vi "CityPinYin.vi"() -> ()   [LabVIEW 2017]
panel:
  out "字符串":string
  out "元素":i32
  out "数组":string[][](array[string])
  out "数据":string
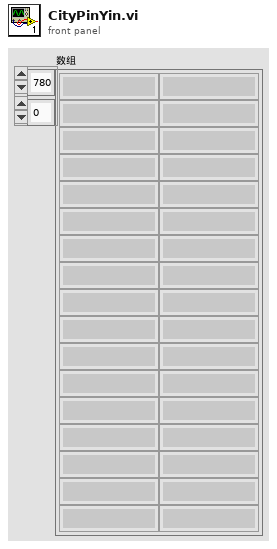
[diagram p1: front panel]
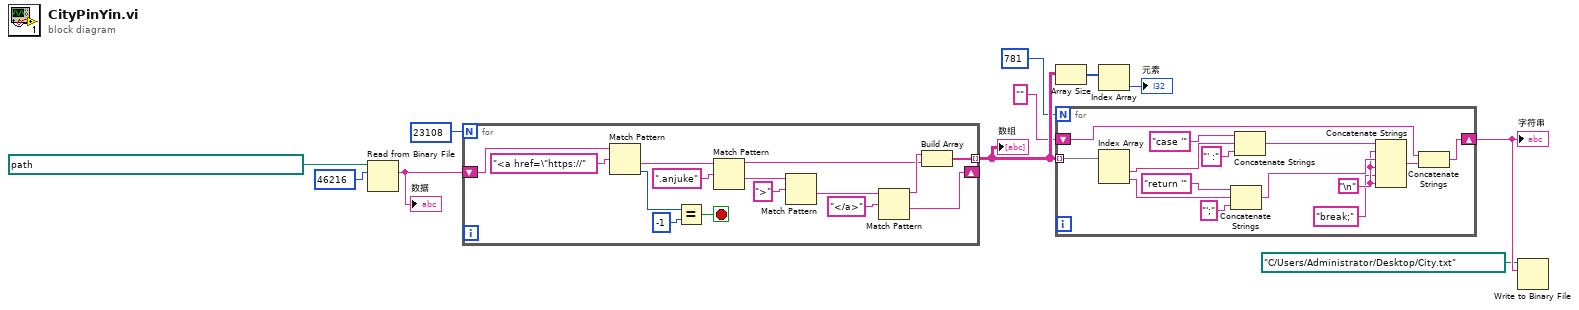
[diagram p0: block diagram]
diagram:
  n1 = Read from Binary File(10:46216 ("总数(1)"), 11:path "C:/Users/Administrator/Desktop/新建文本文档.txt" ("file path (dialog if empty)")) -> (2:w9:string)  [unwired: 4 in, 3 out]
  "数据" <- w9
  n2 = for {
    N: 23108 ("总数(1)") -> [_]
    shift-right: [w18] -> _
    shift-left: w9 -> [w26]
    tunnel: [w15] -> w5 mode=indexing
    stop <- w12 stop-if-true
    n3 = Match Pattern(string=w26, regular expression="<a href=\"https://" ("正则表达式")) -> (after substring=w24:string, offset past match=w14:i32)  [unwired: 1 in, 2 out]
    n4 = Equal?(x=w14, y=-1) -> (x = y?=w12:bool)
    n5 = Match Pattern(string=w24, regular expression=".anjuke" ("正则表达式")) -> (before substring=w16:string, after substring=w22:string)  [unwired: 1 in, 2 out]
    n6 = Match Pattern(string=w22, regular expression=">" ("正则表达式")) -> (after substring=w20:string)  [unwired: 1 in, 3 out]
    n7 = Match Pattern(string=w20, regular expression="</a>" ("正则表达式")) -> (before substring=w17:string, after substring=w18:string)  [unwired: 1 in, 2 out]
    n8 = Build Array(w17, w16) -> (w15:string[])
  }
  "数组" <- w5
  n9 = Array Size(array=w5) -> (size(s)=w7:i32[])
  n10 = for {
    N: 781 -> [_]
    tunnel: w5 -> [w40] mode=indexing
    shift-right: [w29] -> w3
    shift-left: "" -> [w31]
    w28 = "\n"
    n11 = Index Array(array=w40) -> (element #1=w38:string, element #2=w33:string)  [unwired: 2 in]
    n12 = Concatenate Strings("return '", w33, "';" ("字符串")) -> (w32:string)
    n13 = Concatenate Strings("case '", w38, "' :" ("字符串")) -> (w36:string)
    n14 = Concatenate Strings(w36, w28, w32, w28, "break;" ("字符串"), w28) -> (w30:string)
    n15 = Concatenate Strings(w31, w30) -> (w29:string)
  }
  "字符串" <- w3
  n16 = Index Array(array=w7) -> (element=→"元素":i32)  [unwired: 1 in]
  n17 = Write to Binary File(file (use dialog)=path "C:/Users/Administrator/Desktop/City.txt" ("file path (dialog if empty)"), data=w3) -> ()  [unwired: 4 in, 3 out]
